vi "Main Application Instance VIs.vi"(8 "Error In":errorcluster) -> (0 "Error Out":errorcluster)   [LabVIEW 2017, in "Tests.lvlib" / "Bookmark Manager.lvlib"]
uses:
  Bookmark Manager.lvlib
  <vilib>/addons/_JKI Toolkits/Caraya/classes/Test/Test.lvclass
  src/Bookmark Manager/Bookmark Manager.lvlib
  <vilib>/addons/_JKI Toolkits/Caraya/classes/Assert/Assert.lvclass
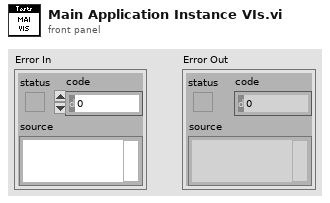
[diagram p1: front panel]
types:
  T1 = typedef "Bookmark Manager.lvlib/VI Information.ctl" = cluster{"App Info":T2, "Name":string, "Path":path}
  T2 = typedef "Bookmark Manager.lvlib/Application Information.ctl" = cluster{"Project":string, "Target":string}
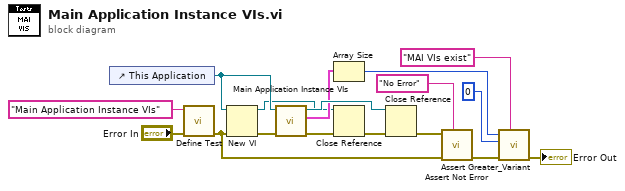
[diagram p0: block diagram]
diagram:
  n1 = control-ref of="This Application"() -> (w3:refnum<vi>)
  n2 = call <vilib>:"Define Test.vi"("error in (no error)"="Error In", "Label (VI Title)"="Main Application Instance VIs") -> ("error out"=w5:errorcluster)  [unwired: 9 in]
  n3 = New VI(8:w5, 11:w3) -> (0:w4:errorcluster, 3:w1:refnum<vi>)  [unwired: 5 in]
  n4 = call "Main Application Instance VIs.vi"("Error In"=w4, "App In"=w3) -> ("Error Out"=w14:errorcluster, "VIs"=w9:T1[], "App Out"=w15:refnum<vi>)  [unwired: 7 in]
  n5 = Array Size(array=w9) -> (size(s)=w8:i32)
  n6 = Close Reference(reference=w1, error in (no error)=w14) -> (error out=w2:errorcluster)
  n7 = Close Reference(reference=w15, error in (no error)=w2) -> (error out=w13:errorcluster)
  n8 = call <vilib>:"Assert Not Error.vi"("Label"="No Error", "error in (no error)"=w5, "Not Error?"=w13) -> ("error out"=w11:errorcluster)  [unwired: 8 in]
  n9 = call <vilib>:"Assert Greater_Variant.vi"("Label"="MAI VIs exist", "error in (no error)"=w11, "Y"=0, "X"=w8) -> ("error out"=→"Error Out":errorcluster)  [unwired: 7 in]
